vi "Receive Message.vi"(8 "error in (no error)":errorcluster, 9 "Mail Strategy In":refnum<class "Mail Strategy.lvclass">, 10 "Wait(ms)":i32=-1, 11 "Messenger Composite in":refnum<class "Tree-ArrayLocation Queue Messenger.lvclass">) -> (0 "error out":errorcluster, 1 "Valid":bool, 2 "Message Out":refnum<class "Message.lvclass">, 3 "Messenger Composite out":refnum<class "Tree-ArrayLocation Queue Messenger.lvclass">)   [LabVIEW 2019, in "Tree-ArrayLocation Queue Messenger.lvclass"]
uses:
  Tree-ArrayLocation Queue Messenger.lvclass
  C:/Users/iio/Desktop/NTHU Brain Center/General Purpose/Classes/Ancestor/Messenger/Messenger Composite/Messenger Composite.lvclass
  Ancestor Class/Message/Message.lvclass
  Ancestor Class/Messenger/Mail Strategy/Mail Strategy.lvclass
  Array Location Mailman/Array Location Mailman.lvclass
  C:/Users/iio/Desktop/NTHU Brain Center/General Purpose/Classes/Ancestor/Messenger/Mail Strategy/Mail Strategy.lvclass
  Array Location Mailman/Array Location Mailman.lvclass/Array Location Mailman.ctl
  Ancestor Class/Messenger/Messenger Composite/Messenger Composite.lvclass/Messenger Composite.ctl
  Tree-ArrayLocation Queue Messenger.lvclass/Tree-ArrayLocation Queue Messenger.ctl
  Array Location Mailman/Public Data/Write Location.vi
  Array Location Mailman/Public Data/Read Location.vi
  Ancestor Class/Messenger/Messenger Composite/Public Data/Read Nodes.vi
  Ancestor Class/Messenger/Messenger/Messenger.lvclass
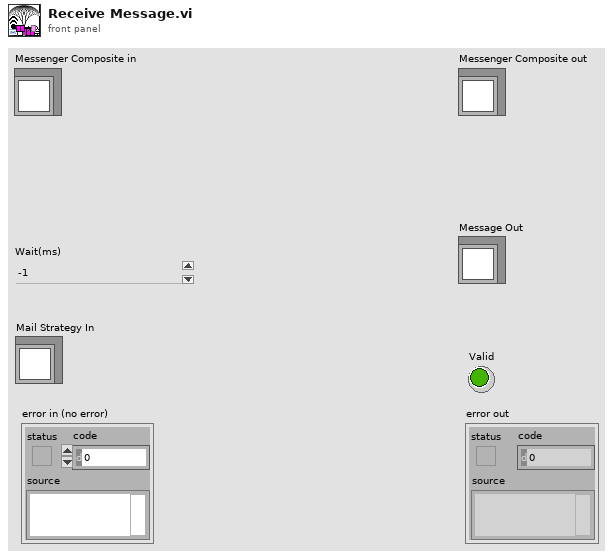
[diagram p1: front panel]
types:
  T1 = typedef "Message Queue.ctl" = refnum<queue>
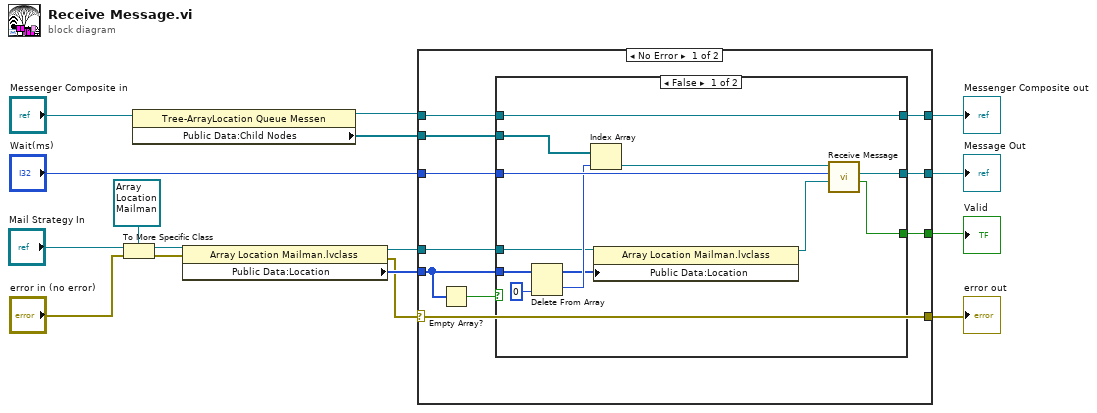
[diagram p0: block diagram]
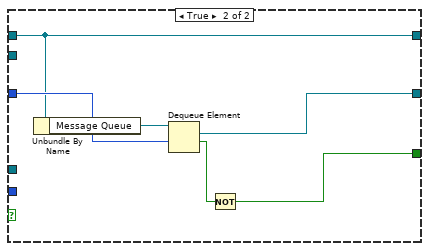
[diagram p2: hidden frame]
diagram:
  n1 = To More Specific Class(target class=refnum<class "Array Location Mailman.lvclass"> refnum ("Array Location Mailman.lvclass"), reference="Mail Strategy In", error in="error in (no error)") -> (specific class reference=w9:refnum<class "Array Location Mailman.lvclass">, error out=w10:errorcluster)
  n2 = property class="Tree-ArrayLocation Queue Messen"(reference="Messenger Composite in") -> (reference out=w2:refnum<class "Tree-ArrayLocation Queue Messenger.lvclass">, "Public Data:Child Nodes"=w1:refnum<class "Messenger.lvclass">[])  [unwired: 1 in, 1 out]
  n3 = property class="Array Location Mailman.lvclass"(reference=w9, error in=w10) -> (reference out=w4:refnum<class "Array Location Mailman.lvclass">, error out=w7:errorcluster, "Public Data:Location"=w8:i32[])
  n4 = case shown="No Error" w7 {
    selector: w7 -> [w24 w46]
    tunnel: w2 -> [w23 w45]
    tunnel: "Wait(ms)" -> [w26 _]
    tunnel: [w25 _] -> w15
    tunnel: [w24 w46] -> w14
    tunnel: [w20 w45] -> w13
    tunnel: [w22 _] -> w12
    tunnel: w8 -> [w19 _]
    tunnel: w4 -> [w18 _]
    tunnel: w1 -> [w17 _]
    frame No Error {
      n5 = Empty Array?(array=w19) -> (empty?=w21:bool)
      n6 = case shown="False" w21 {
        tunnel: w26 -> [w35 w43]
        tunnel: [w33 w42] -> w25
        tunnel: w23 -> [w36 w39]
        tunnel: [w32 w40] -> w22
        tunnel: [w36 w39] -> w20
        tunnel: w19 -> [w38 _]
        tunnel: w18 -> [w30 _]
        tunnel: w17 -> [w27 _]
        frame False {
          n7 = Delete From Array(array=w38, index=0) -> (deleted portion=w31:i32, array with subset deleted=w29:i32[])  [unwired: 1 in]
          n8 = Index Array(array=w27, index=w31) -> (element=w34:refnum<class "Messenger.lvclass">)
          n9 = property class="Array Location Mailman.lvclass"(reference=w30, "Public Data:Location"=w29) -> (reference out=w28:refnum<class "Array Location Mailman.lvclass">)  [unwired: 1 in, 1 out]
          n10 = call-dynamic "Receive Message.vi"("Mail Strategy In"=w28, "Wait(ms)"=w35, "Messenger Component in"=w34) -> ("Valid"=w32:bool, "Message Out"=w33:refnum<class "Message.lvclass">)  [unwired: 5 in, 2 out]
        }
        frame True {
          n11 = Unbundle By Name(w39) -> ("Message Queue"=w44:T1)
          n12 = Dequeue Element(queue=w44, timeout in ms (-1)=w43) -> (element=w42:refnum<class "Message.lvclass">, timed out?=w41:bool)  [unwired: 1 in, 2 out]
          n13 = Not(x=w41) -> (.not. x?=w40:bool)
        }
      }
    }
    frame Error {
    }
  }
  "Messenger Composite out" <- w13
  "Message Out" <- w15
  "Valid" <- w12
  "error out" <- w14
